vi "Cxns-Read Configuration.vi"(0 "Connection File Path":path, 2 "Section":string, 7 "Outputs":string[](array[string]), 11 "error in (no error)":errorcluster) -> (8 "Endpoints":string[](array[string]), 15 "error out":errorcluster)   [LabVIEW 2020]
uses:
  <vilib>/Utility/config.llb/Read Key (String).vi
  <vilib>/Utility/config.llb/NI_LVConfig.lvlib
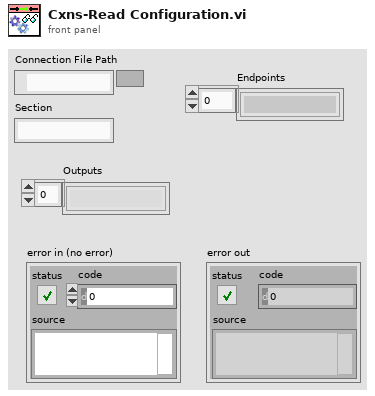
[diagram p1: front panel]
types:
  T1 = typedef "NI_LVConfig.lvlib/Config Data RefNum.ctl" = refnum<k1>
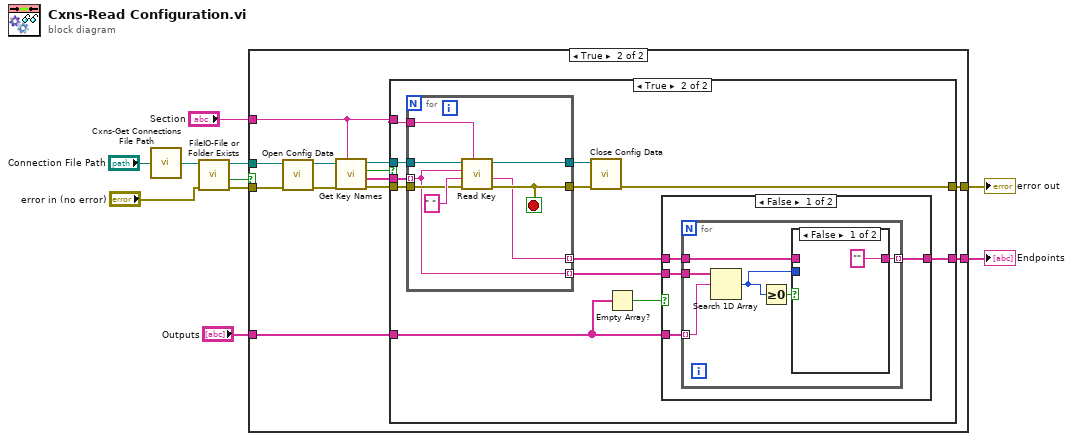
[diagram p0: block diagram]
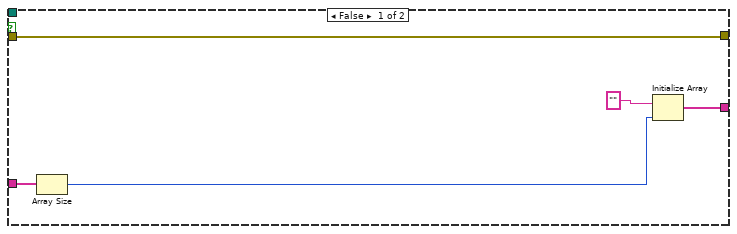
[diagram p2: hidden frame]
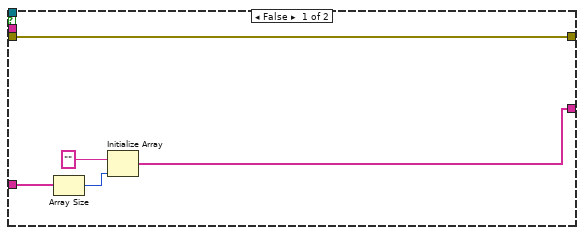
[diagram p3: hidden frame]
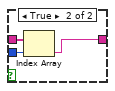
[diagram p4: hidden frame]
diagram:
  n1 = call "Cxns-Get Connections File Path.vi"("Connection File Path"="Connection File Path") -> ("Path Out"=w9:path)
  n2 = call "FileIO-File or Folder Exists.vi"("error in (no error)"="error in (no error)", "path"=w9) -> ("error out"=w5:errorcluster, "Exists?"=w7:bool, "dup path"=w6:path)  [unwired: 6 in, 1 out]
  n3 = case shown="True" w7 {
    tunnel: w6 -> [_ w27]
    tunnel: w5 -> [w15 w26]
    tunnel: "Section" -> [_ w21]
    tunnel: [w15 w19] -> w3
    tunnel: "Outputs" -> [w13 w17]
    tunnel: [w11 w18] -> w1
    frame False {
      n4 = Array Size(array=w13) -> (size(s)=w12:i32)
      n5 = Initialize Array("", w12) -> (w11:string[])
    }
    frame True {
      n6 = call <vilib>:"Open Config Data.vi"("error in (no error)"=w26, "configuration file path"=w27) -> ("error out"=w24:errorcluster, "refnum"=w25:T1)  [unwired: 7 in, 1 out]
      n7 = call <vilib>:"Get Key Names.vi"("section"=w21, "error in (no error)"=w24, "refnum"=w25) -> ("error out"=w20:errorcluster, "key names"=w22:string[], "section exists?"=w16:bool, "refnum out"=w23:T1)  [unwired: 5 in]
      n8 = case shown="True" w16 {
        tunnel: w23 -> [_ w44]
        tunnel: w22 -> [_ w43]
        tunnel: w21 -> [_ w42]
        tunnel: w20 -> [w28 w41]
        tunnel: [w28 w38] -> w19
        tunnel: [w29 w35] -> w18
        tunnel: w17 -> [w30 w33]
        frame False {
          n9 = Array Size(array=w30) -> (size(s)=w32:i32)
          n10 = Initialize Array("", w32) -> (w29:string[])
        }
        frame True {
          n11 = for {
            tunnel: w44 -> [w67]
            tunnel: w43 -> [w61] mode=indexing
            tunnel: [w65] -> w39
            tunnel: w42 -> [w64]
            tunnel: [w60] -> w37 mode=indexing
            tunnel: w41 -> [w63]
            tunnel: [w62] -> w40
            tunnel: [w61] -> w34 mode=indexing
            stop <- w62 stop-if-true
            n12 = call-poly <vilib>:"Read Key.vi"("section"=w64, "error in (no error)"=w63, "default value"=" ", "key"=w61, "refnum"=w67) -> ("error out"=w62:errorcluster, "value"=w60:string, "refnum out"=w65:T1)  [unwired: 3 in, 1 out]
          }
          n13 = call <vilib>:"Close Config Data.vi"("error in (no error)"=w40, "refnum"=w39) -> ("error out"=w38:errorcluster)  [unwired: 8 in, 1 out]
          n14 = Empty Array?(array=w33) -> (empty?=w36:bool)
          n15 = case shown="False" w36 {
            tunnel: w37 -> [w46 w59]
            tunnel: [w45 w59] -> w35
            tunnel: w34 -> [w47 _]
            tunnel: w33 -> [w48 _]
            frame False {
              n16 = for {
                tunnel: w48 -> [w49] mode=indexing
                tunnel: w47 -> [w54]
                tunnel: w46 -> [w53]
                tunnel: [w52] -> w45 mode=indexing
                n17 = Search 1D Array(1D array=w54, element=w49) -> (index of element=w51:i32)  [unwired: 1 in]
                n18 = Greater Or Equal To 0?(x=w51) -> (x >= 0?=w50:bool)
                n19 = case shown="False" w50 {
                  tunnel: w53 -> [_ w58]
                  tunnel: ["" w57] -> w52
                  tunnel: w51 -> [_ w56]
                  frame False {
                  }
                  frame True {
                    n20 = Index Array(array=w58, index=w56) -> (element=w57:string)
                  }
                }
              }
            }
            frame True {
            }
          }
        }
      }
    }
  }
  "error out" <- w3
  "Endpoints" <- w1
